vi "weed.vi"(8 "picture":picture, 9 "color":i16, 10 "y":dbl, 11 "x":dbl) -> (3 "new picture":picture)   [LabVIEW 2016]
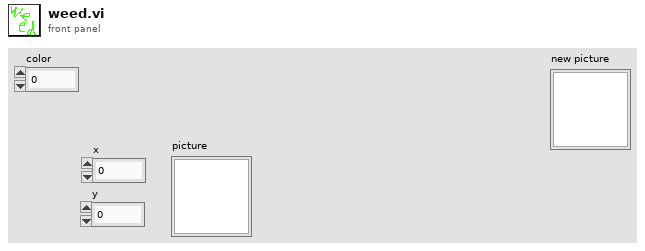
[diagram p1: front panel]
types:
  T1 = cluster{"Width":u16, "Style":enum32{"Solid", "Dash", "Dot", "DashDot", "DashDotDot"}}
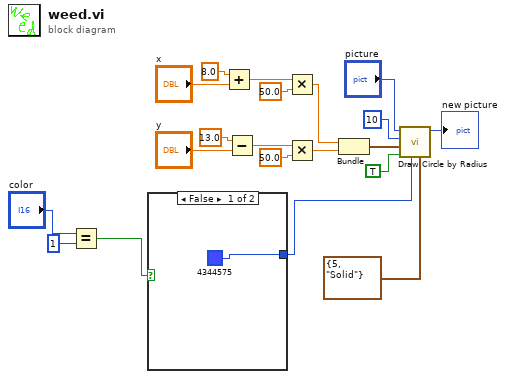
[diagram p0: block diagram]
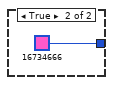
[diagram p2: hidden frame]
diagram:
  n1 = Equal?(x="color", y=i16 1) -> (x = y?=w2:bool)
  n2 = case shown="False" w2 {
    tunnel: [u32 4344575 ("color(black)") u32 16734666 ("color(black)")] -> w1
    frame False {
    }
    frame True {
    }
  }
  n3 = Add(x=8.0, y="x") -> (x+y=w11:dbl)
  n4 = Subtract(x=13.0 ("y"), y="y") -> (x-y=w10:dbl)
  n5 = Multiply(x=w11, y=50.0) -> (x*y=w8:dbl)
  n6 = Multiply(x=w10, y=50.0) -> (x*y=w7:dbl)
  n7 = Bundle(w8, w7) -> (w15:cluster{dbl, dbl})  [unwired: 1 in]
  n8 = call <vilib>:"Draw Circle by Radius.vi"("pen"=T1 {"Width"=5, "Style"=enum."Solid"}, "color(black)"=w1, "fill?(F)"=TRUE, "pixel center"=w15, "radius"=i16 10, "picture"="picture") -> ("new picture"=→"new picture":picture)  [unwired: 5 in]
